vi "Senden-2_ECD.vi"(5 "error in":errorcluster, 6 "BefehlsCluster":T1, 7 "AbfragenCluster":cluster{string[], string[], string[]}, 8 "Abfragenr.Cluster":cluster{i32, i32, i32}, 9 "Senden?":bool[](array[boolean]), 10 "FPGA-VI-Referenz":refnum<k20>) -> (0 "BefehlsCluster":T1, 2 "error out":errorcluster, 3 "Senden?":bool[](array[boolean]), 4 "Abfragenr.Cluster":cluster{i32, i32, i32})   [LabVIEW 2017]
uses:
  <vilib>/rvi/interface/nirviMethod/nirviMethod.xnode
  FPGA Bitfiles/HAGAR-VECD_FPGATarget_FPGA-ProgrammECD_J-wKM9Jb3G8.lvbitx
  E:/HAGAR-V_ECD/FPGA-Programm_ECD.vi
  <vilib>/rvi/errors/niLvFpgaMergeErrorWithErrorCode.vi
  <vilib>/FPGAPlugInAG/cRIO-9035/niLvFpga_WriteFifo_cRIO-9035.vi
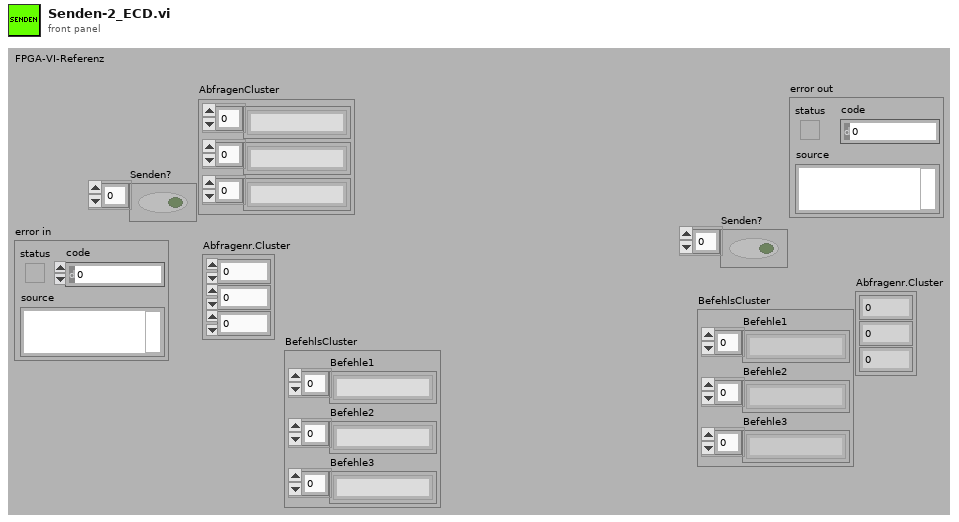
[diagram p1: front panel]
types:
  T1 = cluster{"Befehle1":string[], "Befehle2":string[], "Befehle3":string[]}
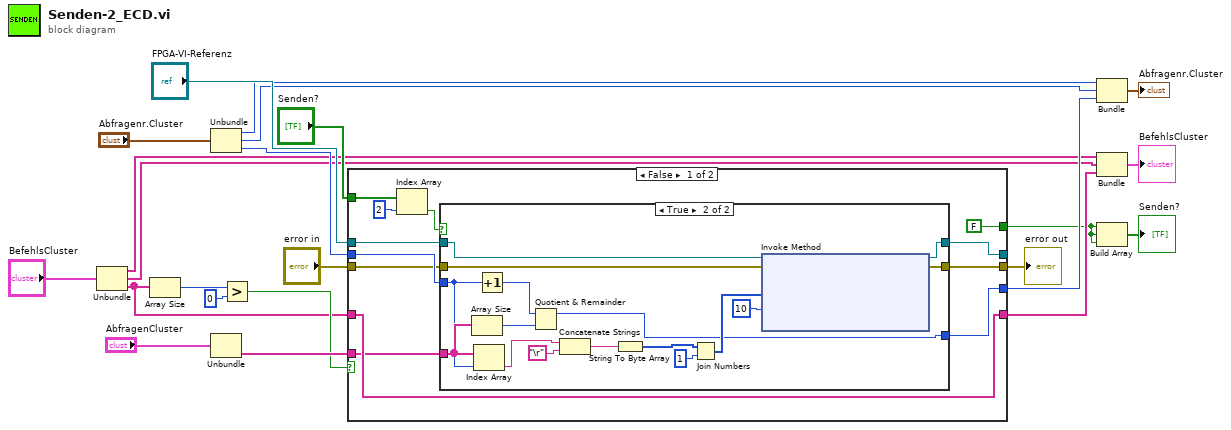
[diagram p0: block diagram]
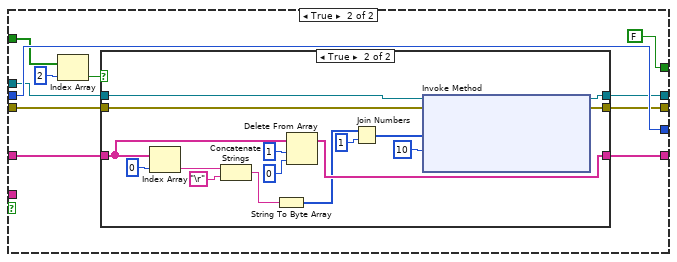
[diagram p3: hidden frame]
diagram:
  n1 = Unbundle("BefehlsCluster") -> ("Befehle1"=w1:string[], "Befehle2"=w2:string[], "Befehle3"=w18:string[])
  n2 = Array Size(array=w18) -> (size(s)=w22:i32)
  n3 = Unbundle("Abfragenr.Cluster") -> (w3:i32, w4:i32, w13:i32)
  n4 = Unbundle("AbfragenCluster") -> (w23:string[])  [unwired: 2 out]
  n5 = Greater?(x=w22, y=0) -> (0:w20:bool)
  n6 = case shown="False" w20 {
    tunnel: w18 -> [w35 w62]
    tunnel: [w35 w61] -> w17
    tunnel: "Senden?" -> [w29 w59]
    tunnel: w13 -> [w32 w65]
    tunnel: "FPGA-VI-Referenz" -> [w31 w60]
    tunnel: [w30 w65] -> w12
    tunnel: w23 -> [w28 _]
    tunnel: [FALSE FALSE] -> w6
    tunnel: [w26 w57] -> _
    tunnel: "error in" -> [w25 w56]
    tunnel: [w24 w55] -> w8
    frame False {
      n7 = Index Array(array=w29, index=2 ("Index")) -> (element=w33:bool)
      n8 = case shown="True" w33 {
        tunnel: w28 -> [_ w52]
        tunnel: w32 -> [w38 w46]
        tunnel: w31 -> [w37 w49]
        tunnel: [w38 w45] -> w30
        tunnel: [w37 w44] -> w26
        tunnel: w25 -> [w36 w40]
        tunnel: [w36 w39] -> w24
        frame False {
        }
        frame True {
          n9 = Array Size(array=w52) -> (size(s)=w53:i32)
          n10 = Index Array(array=w52, index=w46) -> (element=w42:string)
          n11 = Increment(x=w46) -> (x+1=w54:i32)
          n12 = Quotient & Remainder(x=w54, y=w53) -> (x-y*floor(x/y)=w45:i32)  [unwired: 1 out]
          n13 = Concatenate Strings(w42, "\r") -> (w41:string)
          n14 = String To Byte Array(string=w41) -> (unsigned byte array=w51:u8[])
          n15 = Join Numbers(hi=w51, lo=u8 1) -> ((hi.lo)=w48:u16[])
          n16 = xnode "Invoke Method"("FPGA-VI-Referenz (Eingang)"=w49, "Fehler (Eingang)"=w40, "Daten"=w48, "Timeout (ms)"=10) -> ("FPGA-VI-Referenz (Ausgang)"=w44:refnum<k20>, "Fehler (Ausgang)"=w39:errorcluster)  [unwired: 1 out]
        }
      }
    }
    frame True {
      n17 = Index Array(array=w59, index=2 ("Index")) -> (element=w63:bool)
      n18 = case shown="True" w63 {
        tunnel: w62 -> [w68 w80]
        tunnel: [w68 w82] -> w61
        tunnel: w60 -> [w67 w81]
        tunnel: [w67 w74] -> w57
        tunnel: w56 -> [w66 w70]
        tunnel: [w66 w69] -> w55
        frame False {
        }
        frame True {
          n19 = Index Array(array=w80, index=0 ("Index")) -> (element=w72:string)
          n20 = Concatenate Strings(w72, "\r") -> (w71:string)
          n21 = String To Byte Array(string=w71) -> (unsigned byte array=w78:u8[])
          n22 = Delete From Array(array=w80, length=1 ("Länge"), index=0 ("Index")) -> (array with subset deleted=w82:string[])  [unwired: 1 out]
          n23 = Join Numbers(hi=w78, lo=u8 1) -> ((hi.lo)=w76:u16[])
          n24 = xnode "Invoke Method"("FPGA-VI-Referenz (Eingang)"=w81, "Fehler (Eingang)"=w70, "Daten"=w76, "Timeout (ms)"=10) -> ("FPGA-VI-Referenz (Ausgang)"=w74:refnum<k20>, "Fehler (Ausgang)"=w69:errorcluster)  [unwired: 1 out]
        }
      }
    }
  }
  "error out" <- w8
  n25 = Bundle(w3, w4, w12) -> (→"Abfragenr.Cluster":cluster{i32, i32, i32})  [unwired: 1 in]
  n26 = Bundle("Befehle1"=w1, "Befehle2"=w2, "Befehle3"=w17) -> (→"BefehlsCluster":T1)  [unwired: 1 in]
  n27 = Build Array(w6, w6, w6) -> (→"Senden?":bool[])
